vi "Write Settings.vi"(8 "error in (no error)":errorcluster, 9 "Channel":string, 10 "Settings":T1={"Dt"=0.002, "#samples"=10000, "t0"=0.0} {"Dt" format="%.2e"}, 11 "Agilent DSO-X 3032A in":refnum<class "Agilent DSO-X 3032A.lvclass">) -> (0 "error out":errorcluster, 3 "Agilent DSO-X 3032A out":refnum<class "Agilent DSO-X 3032A.lvclass">)   [LabVIEW 2014, in "Agilent DSO-X 3032A.lvclass"]
uses:
  Agilent DSO-X 3032A.lvclass
  Channel Settings.ctl
  Agilent DSO-X 3032A.lvclass/Agilent DSO-X 3032A.ctl
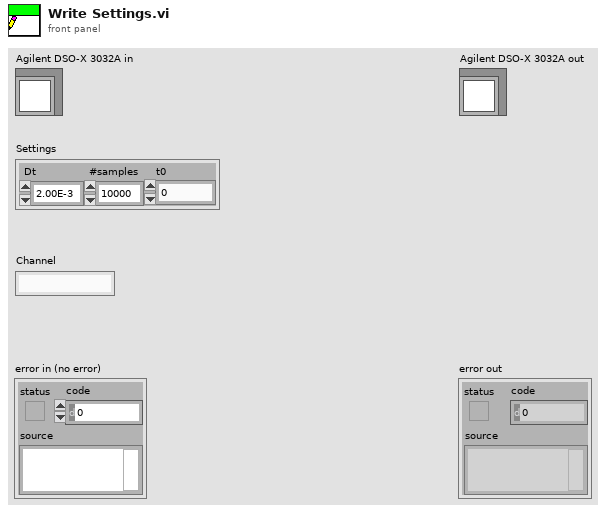
[diagram p1: front panel]
types:
  T1 = typedef "Agilent DSO-X 3032A.lvclass/Channel Settings.ctl" = cluster{"Dt":dbl, "#samples":i32, "t0":dbl}
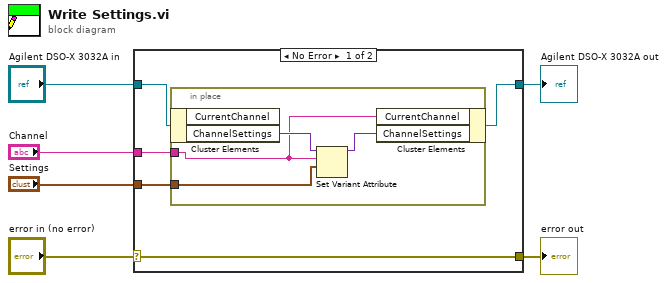
[diagram p0: block diagram]
diagram:
  n1 = case shown="No Error" "error in (no error)" {
    selector: "error in (no error)" -> [w11 w16]
    tunnel: [w11 w16] -> w5
    tunnel: [w9 w17] -> w3
    tunnel: "Agilent DSO-X 3032A in" -> [w10 w17]
    tunnel: "Settings" -> [w7 _]
    tunnel: "Channel" -> [w8 _]
    frame No Error {
      n2 = in-place {
        in-place-border: w8 -> [w12]
        in-place-border: w7 -> [w13]
        n3 = in-place-cluster #1(w10) -> ("ChannelSettings"=w15:variant)  [unwired: 1 out]
        n4 = Set Variant Attribute(Variant=w15, name=w12, value=w13) -> (Variant out=w14:variant)  [unwired: 1 in, 2 out]
        n5 = in-place-cluster #1("CurrentChannel"=w12, "ChannelSettings"=w14) -> (w9:refnum<class "Agilent DSO-X 3032A.lvclass">)
      }
    }
    frame Error {
    }
  }
  "error out" <- w5
  "Agilent DSO-X 3032A out" <- w3
